vi "Rec_organize data_2.vi"(7 "write mode":enum16{"XYZ", "XYZ_err", "Z"}(ring), 9 "beads track":T1[](array[typedef]) {"centroid"."Y Centroid" format="%.2f"; "centroid"."X Centroid" format="%.2f"; "ROI Des out"."Contours"."Type" items=["No Selection", "Point", "Line", "Rectangle", "Oval", "Polygon", "Freehand Region", "Annulus", "Unused2", "Unused3", "Broken Line", "Freehand Line", "Rotated Rectangle"]}) -> (2 "rec array":dbl[][][](array[numeric]))   [LabVIEW 2017]
doc: "本VI的作用是将分析循环得出的XYZ信息，以及当前的磁铁位置信息，按照磁球序号进行重新组织，方便写入TDMS文件，组织顺序和创建的通道顺序一致。\n组织过程中可以选取一个磁球作为参考球，但也可以选择不要参考球。"
uses:
  control/Bead track.ctl
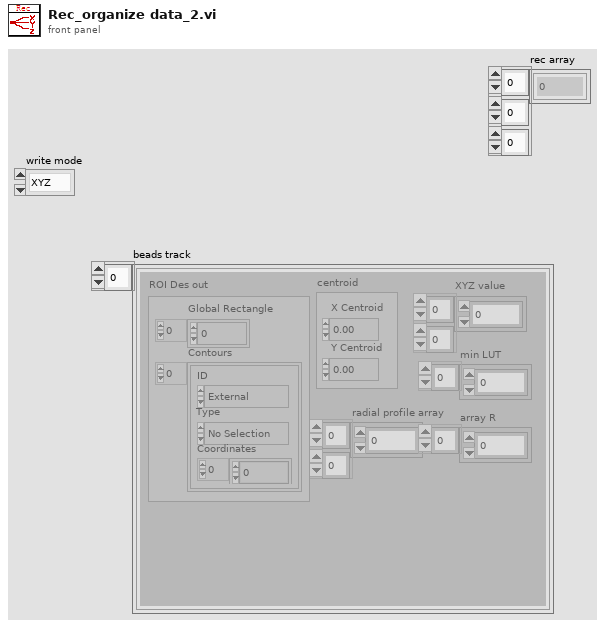
[diagram p1: front panel]
types:
  T1 = typedef "Bead track.ctl" = cluster{"XYZ value":dbl[][], "radial profile array":dbl[][], "min LUT":dbl[], "ROI Des out":T2, "array R":dbl[], "centroid":cluster{"X Centroid":sgl, "Y Centroid":sgl}}
  T2 = typedef "ROI Descriptor" = cluster{"Global Rectangle":i32[], "Contours":cluster{"ID":enum32{"External", "Internal"}, "Type":u32, "Coordinates":i32[]}[]}
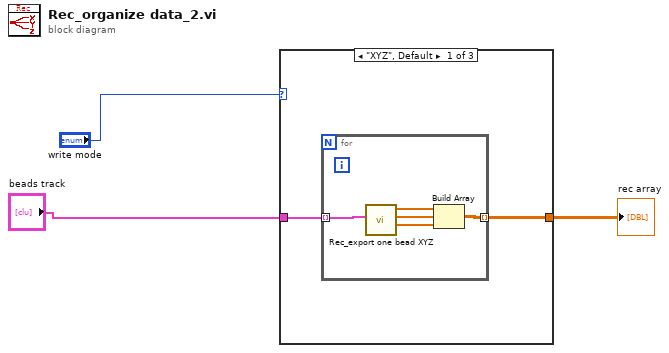
[diagram p0: block diagram]
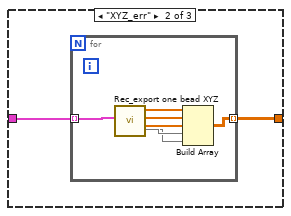
[diagram p2: hidden frame]
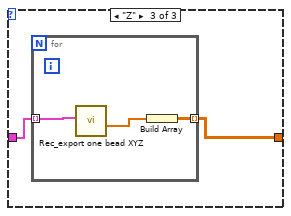
[diagram p3: hidden frame]
diagram:
  n1 = case shown="\"XYZ\", Default" "write mode" {
    tunnel: "beads track" -> [w5 w12 w21]
    tunnel: [w4 w11 w20] -> w2
    frame "XYZ", Default {
      n2 = for {
        tunnel: w5 -> [w7] mode=indexing
        tunnel: [w6] -> w4 mode=indexing
        n3 = call "Rec_export one bead XYZ.vi"("beads track"=w7) -> ("Z"=w8:dbl[], "Y"=w9:dbl[], "X"=w10:dbl[])  [unwired: 8 in]
        n4 = Build Array(w10, w9, w8) -> (w6:dbl[][])
      }
    }
    frame "XYZ_err" {
      n5 = for {
        tunnel: w12 -> [w16] mode=indexing
        tunnel: [w15] -> w11 mode=indexing
        n6 = call "Rec_export one bead XYZ.vi"("beads track"=w16) -> ("Z"=w17:dbl[], "Y"=w18:dbl[], "X"=w19:dbl[], 4:w13, 6:w14)  [unwired: 6 in]
        n7 = Build Array(w19, w18, w17, w14, w13) -> (w15:dbl[][])
      }
    }
    frame "Z" {
      n8 = for {
        tunnel: w21 -> [w23] mode=indexing
        tunnel: [w22] -> w20 mode=indexing
        n9 = call "Rec_export one bead XYZ.vi"("beads track"=w23) -> ("Z"=w24:dbl[])  [unwired: 8 in, 2 out]
        n10 = Build Array(w24) -> (w22:dbl[][])
      }
    }
  }
  "rec array" <- w2
